vi "Place HDI Precheck.vi"(8 "error in":errorcluster, 9 "Slot Number in":i32, 10 "Chuck Number in":i32, 11 "PickupTool Class in":refnum<class "PickerTool Class.lvclass">) -> (0 "error out":errorcluster, 3 "PickupTool Class out":refnum<class "PickerTool Class.lvclass">)   [LabVIEW 2011, in "PickerTool Class.lvclass"]
uses:
  PickerTool Class.lvclass
  PickerTool Class.lvclass/PickerTool Class.ctl
  WorkTable Class/WorkTable Class.lvclass
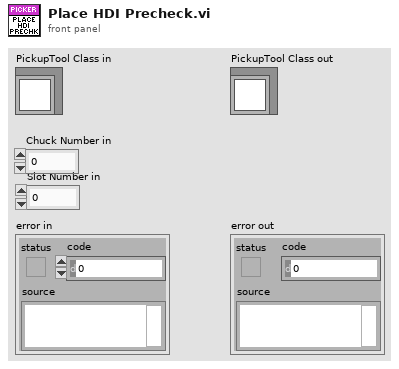
[diagram p1: front panel]
types:
  T1 = typedef "Worktable_Module Slot.ctl" = cluster{"Slot State":enum16{"Empty", "Bare HDI", "Unglued", "Stamped", "PartOnTop", "Weighted", "Unpotted", "Potted"}, "BBM Type":enum16{"None", "BBM", "GlassSlide"}, "HDI Type":enum16{"None", "HDI", "Polyimide"}, "Vacuum Channel":u8, "Location/Orientation BBM":T2, "Location/Orientation HDI":T2, "S/N":string}
  T2 = typedef "Position_Orientation.ctl" = cluster{"Center":refnum<class "Vec3d Class.lvclass">, "Orientation":refnum<class "Orient3d Class.lvclass">}
  T3 = enum16{"Empty", "Bare HDI", "Unglued", "Stamped", "PartOnTop", "Weighted", "Unpotted", "Potted"}
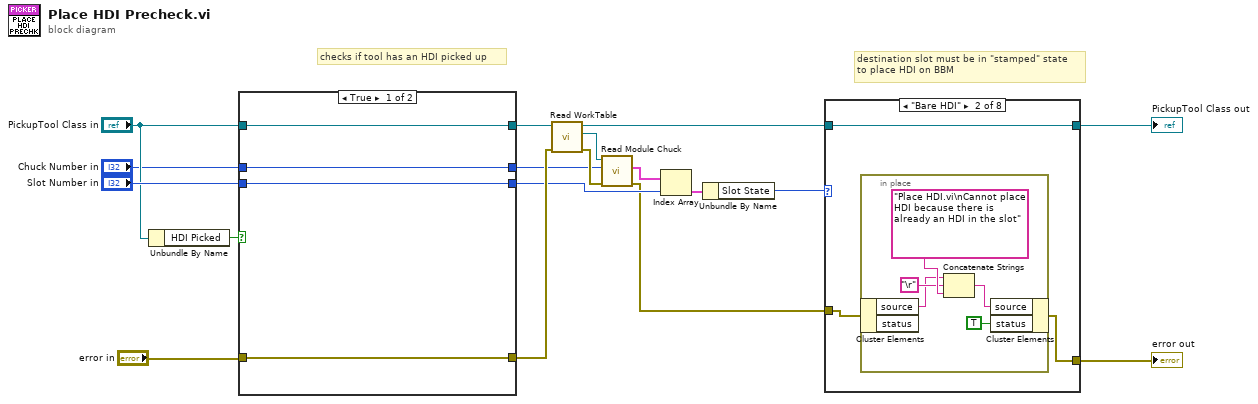
[diagram p0: block diagram]
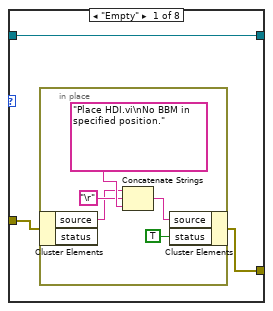
[diagram p2: hidden frame]
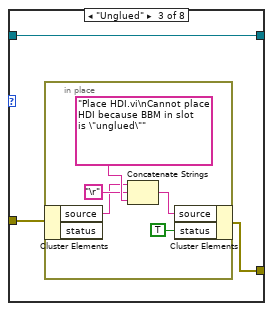
[diagram p3: hidden frame]
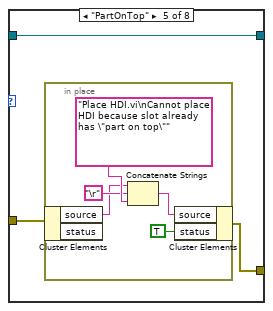
[diagram p5: hidden frame]
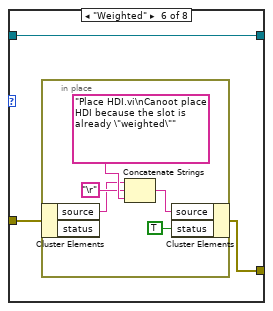
[diagram p6: hidden frame]
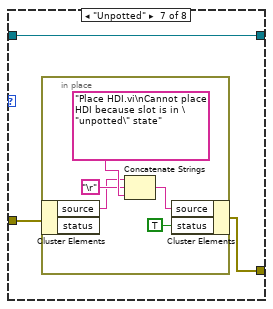
[diagram p7: hidden frame]
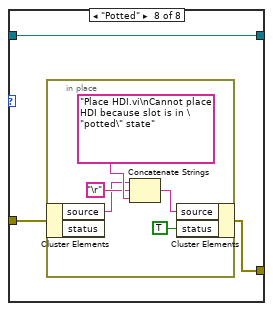
[diagram p8: hidden frame]
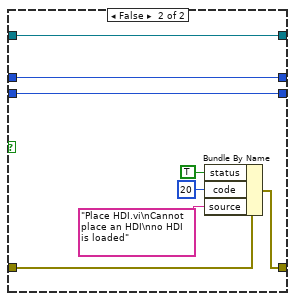
[diagram p9: hidden frame]
diagram:
  # "destination slot must be in \"stamped\" state\nto place HDI on BBM"
  # "checks if tool has an HDI picked up"
  n1 = Unbundle By Name("PickupTool Class in") -> ("HDI Picked"=w12:bool)
  n2 = case shown="True" w12 {
    tunnel: "PickupTool Class in" -> [w22 w30]
    tunnel: "error in" -> [w21 w29]
    tunnel: [w22 w30] -> w14
    tunnel: [w21 w25] -> w15
    tunnel: "Slot Number in" -> [w20 w24]
    tunnel: [w20 w24] -> w5
    tunnel: "Chuck Number in" -> [w19 w23]
    tunnel: [w19 w23] -> w7
    frame True {
    }
    frame False {
      n3 = Bundle By Name(cluster=w29, "status"=TRUE, "code"=20, "source"="Place HDI.vi\nCannot place an HDI\nno HDI is loaded") -> (w25:errorcluster)
    }
  }
  n4 = call-dynamic "Read WorkTable.vi"("error in"=w15, "Gantry Class in"=w14) -> ("error out"=w9:errorcluster, "WorkTable Class.lvclass"=w8:refnum<class "WorkTable Class.lvclass">, "Gantry Class out"=w17:refnum<class "PickerTool Class.lvclass">)  [unwired: 7 in]
  n5 = call-dynamic "Read Module Chuck.vi"("error in"=w9, "index"=w7, "WorkTable in"=w8) -> ("error out"=w3:errorcluster, "Module Slots"=w6:T1[])  [unwired: 6 in, 1 out]
  n6 = Index Array(array=w6, index=w5) -> (element=w4:T1)
  n7 = Unbundle By Name(w4) -> ("Slot State"=w1:T3)
  n8 = case shown="\"Bare HDI\"" w1 {
    tunnel: w17 -> [w32 w41 w47 w56 w57 w65 w73 w81]
    tunnel: [w33 w40 w49 w55 w59 w67 w75 w83] -> w2
    tunnel: [w32 w41 w47 w56 w57 w65 w73 w81] -> w18
    tunnel: w3 -> [w31 w39 w48 w55 w58 w66 w74 w82]
    frame "Empty" {
      n9 = in-place {
        n10 = in-place-cluster #1(w31) -> ("source"=w35:string)  [unwired: 1 out]
        n11 = Concatenate Strings(w35, "\r", "Place HDI.vi\nNo BBM in specified position." ("string")) -> (w36:string)
        n12 = in-place-cluster #1("source"=w36, "status"=TRUE) -> (w33:errorcluster)
      }
    }
    frame "Bare HDI" {
      n13 = in-place {
        n14 = in-place-cluster #2(w39) -> ("source"=w43:string)  [unwired: 1 out]
        n15 = Concatenate Strings(w43, "\r", "Place HDI.vi\nCannot place HDI because there is already an HDI in the slot" ("string")) -> (w44:string)
        n16 = in-place-cluster #2("source"=w44, "status"=TRUE) -> (w40:errorcluster)
      }
    }
    frame "Unglued" {
      n17 = in-place {
        n18 = in-place-cluster #3(w48) -> ("source"=w51:string)  [unwired: 1 out]
        n19 = Concatenate Strings(w51, "\r", "Place HDI.vi\nCannot place HDI because BBM in slot is \"unglued\"" ("string")) -> (w52:string)
        n20 = in-place-cluster #3("source"=w52, "status"=TRUE) -> (w49:errorcluster)
      }
    }
    frame "Stamped" {
    }
    frame "PartOnTop" {
      n21 = in-place {
        n22 = in-place-cluster #4(w58) -> ("source"=w61:string)  [unwired: 1 out]
        n23 = Concatenate Strings(w61, "\r", "Place HDI.vi\nCannot place HDI because slot already has \"part on top\"" ("string")) -> (w62:string)
        n24 = in-place-cluster #4("source"=w62, "status"=TRUE) -> (w59:errorcluster)
      }
    }
    frame "Weighted" {
      n25 = in-place {
        n26 = in-place-cluster #5(w66) -> ("source"=w69:string)  [unwired: 1 out]
        n27 = Concatenate Strings(w69, "\r", "Place HDI.vi\nCanoot place HDI because the slot is already \"weighted\"" ("string")) -> (w70:string)
        n28 = in-place-cluster #5("source"=w70, "status"=TRUE) -> (w67:errorcluster)
      }
    }
    frame "Unpotted" {
      n29 = in-place {
        n30 = in-place-cluster #6(w74) -> ("source"=w77:string)  [unwired: 1 out]
        n31 = Concatenate Strings(w77, "\r", "Place HDI.vi\nCannot place HDI because slot is in \"unpotted\" state" ("string")) -> (w78:string)
        n32 = in-place-cluster #6("source"=w78, "status"=TRUE) -> (w75:errorcluster)
      }
    }
    frame "Potted" {
      n33 = in-place {
        n34 = in-place-cluster #7(w82) -> ("source"=w85:string)  [unwired: 1 out]
        n35 = Concatenate Strings(w85, "\r", "Place HDI.vi\nCannot place HDI because slot is in \"potted\" state" ("string")) -> (w86:string)
        n36 = in-place-cluster #7("source"=w86, "status"=TRUE) -> (w83:errorcluster)
      }
    }
  }
  "error out" <- w2
  "PickupTool Class out" <- w18
